vi "Read Single.vi"(8 "error in":errorcluster, 10 "portBit":i32=-1, 11 "task in":i32) -> (0 "error out":errorcluster, 2 "data":u8, 3 "task out":i32)   [LabVIEW 2025, in "DIO.lvlib"]
uses:
  DIO.lvlib
  <userlib>/DAQNavi Polymorphic VI/read/DAQNavi Read (Digital U8 1Chan 1Samp).vi
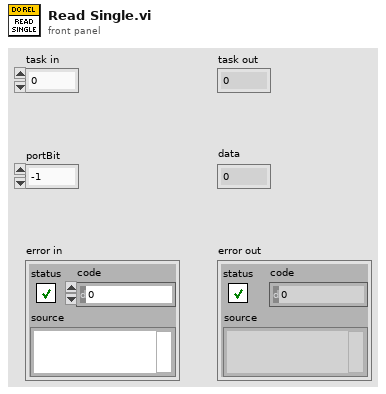
[diagram p1: front panel]
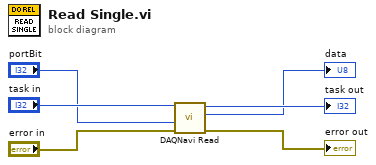
[diagram p0: block diagram]
diagram:
  n1 = call-poly <userlib>:"DAQNavi Read.vi"("error in (no error)"="error in", "portBit"="portBit", "task in"="task in") -> ("error out"=→"error out":errorcluster, "data"=→"data":u8, "task out"=→"task out":i32)  [unwired: 1 in, 5 out]
